vi "Python_Coordinates.vi"(8 "Angle and distance":bool) -> (0 "Coordinates":dbl[][](array[numeric]))   [LabVIEW 2021]
doc: "This example demonstrates how to call a Python function and pass integers as arguments. It uses a python function to compute the sum of two integers."
uses:
  Global_Variables.vi
panel:
  out "error out 2":errorcluster
  in  "error in (no error) 2":errorcluster
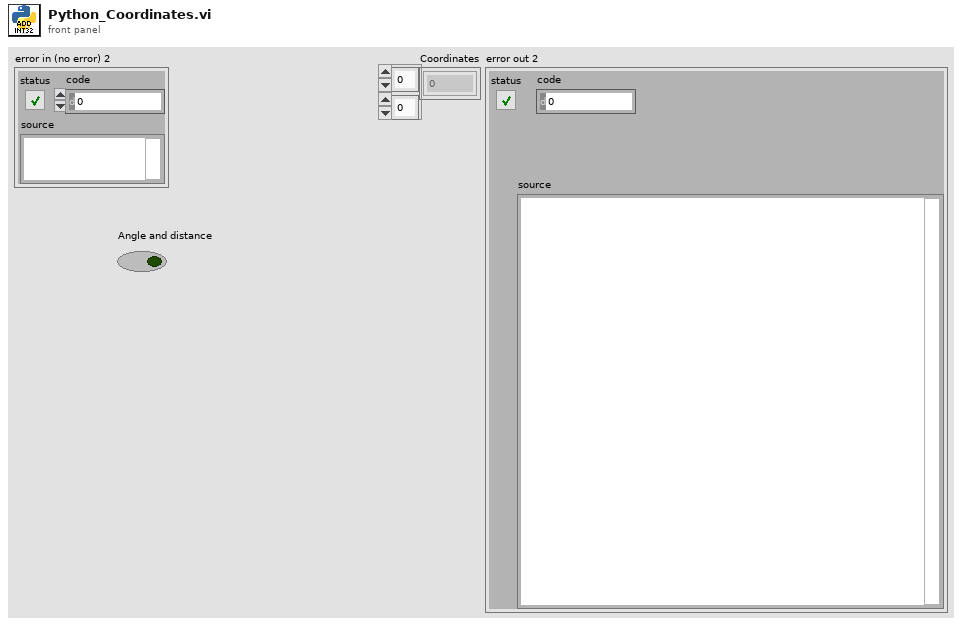
[diagram p1: front panel]
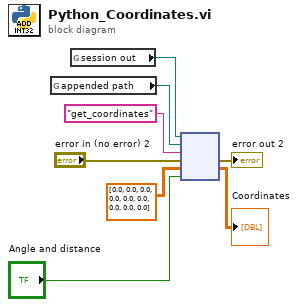
[diagram p0: block diagram]
diagram:
  n1 = global read "Global_Variables.vi" "appended path"() -> (w5:path)
  n2 = global read "Global_Variables.vi" "session out"() -> (w4:refnum<k35>)
  n3 = node(w4, w5, "get_coordinates" ("function name"), "error in (no error) 2", dbl[][] [[0.0, 0.0, 0.0], [0.0, 0.0, 0.0], [0.0, 0.0, 0.0]], "Angle and distance") -> (→"error out 2":errorcluster, →"Coordinates":dbl[][])  [unwired: 1 in, 3 out]
